vi "Write All Control Values.vi"(8 "error in (no error)":errorcluster, 11 "CD Parameter Manager in":refnum<class "CD Parameter Manager.lvclass">) -> (0 "error out":errorcluster, 3 "CD Parameter Manager out":refnum<class "CD Parameter Manager.lvclass">)   [LabVIEW 2019, in "CD Parameter Manager API.lvlib" / "CD Parameter Manager.lvclass"]
uses:
  CD Parameter Manager.lvclass
  CD Parameter Manager.lvclass/CD Parameter Manager.ctl
  Parameter Class/Parameter.lvclass
panel:
  in  "VI Ref":refnum<vi>
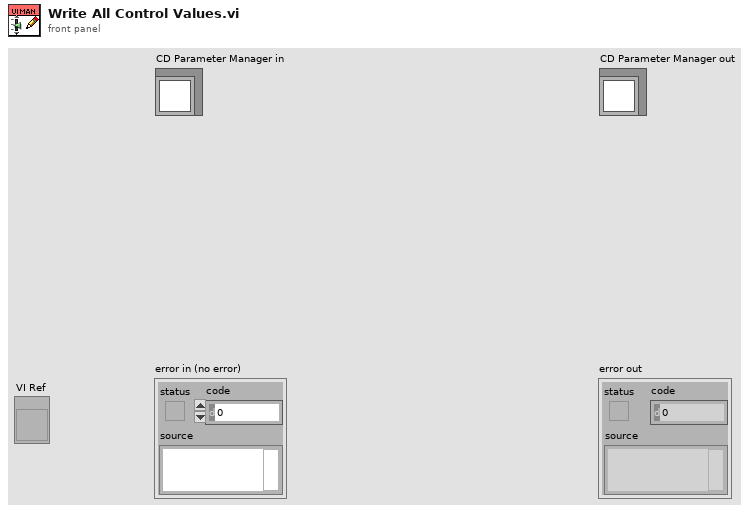
[diagram p1: front panel]
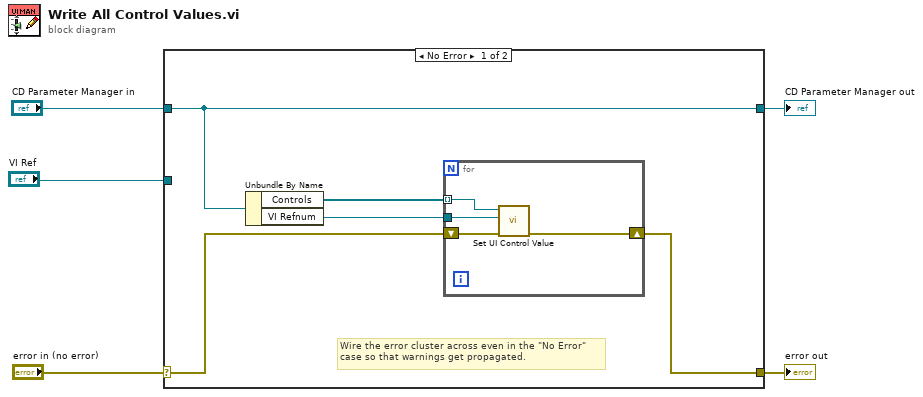
[diagram p0: block diagram]
diagram:
  n1 = case shown="No Error" "error in (no error)" {
    selector: "error in (no error)" -> [w7 w16]
    tunnel: [w6 w16] -> w4
    tunnel: [w10 w15] -> w2
    tunnel: "CD Parameter Manager in" -> [w10 w15]
    tunnel: "VI Ref" -> [_ _]
    frame No Error {
      # "Wire the error cluster across even in the \"No Error\"\ncase so that warnings get propagated."
      n2 = Unbundle By Name(w10) -> ("Controls"=w8:refnum<class "Parameter.lvclass">[], "VI Refnum"=w9:refnum<vi>)
      n3 = for {
        tunnel: w9 -> [w14]
        tunnel: w8 -> [w13] mode=indexing
        shift-right: [w11] -> w6
        shift-left: w7 -> [w12]
        n4 = call-dynamic "Set UI Control Value.vi"("error in (no error)"=w12, "VI Ref"=w14, "Parameter in"=w13) -> ("error out"=w11:errorcluster)  [unwired: 7 in, 1 out]
      }
    }
    frame Error {
    }
  }
  "error out" <- w4
  "CD Parameter Manager out" <- w2
